vi "Test D Datagrid.vi"() -> ()   [LabVIEW 2020]
uses:
  U32 D Element/U32 D Element.lvclass
  C:/dev/D Datagrid/DatagridElement/DatagridElement.lvclass
  Float D Element/Float D Element.lvclass
  Bool D Element/Bool D Element.lvclass
  U32 D Element/Display mode.ctl
  Double D Element/Double D Element.lvclass
  C:/dev/D Datagrid/Floating point base/Floating point base.lvclass
  D_Datagrid.lvclass
  U32 D Element/U32 D Element.lvclass/U32 D Element.ctl
  Floating point base/Floating point base.lvclass/Floating point base.ctl
  D_Datagrid.lvclass/D_Datagrid.ctl
  Floating point base/Write Format string.vi
  U32 D Element/Write Display mode.vi
  Read Auto update indicator.vi
  Redraw full indicator.vi
panel:
  in  "Table Control":string[][](table)
  # "#TODO:\n\n-Make sure all keybinds work correctly (tabs?)"
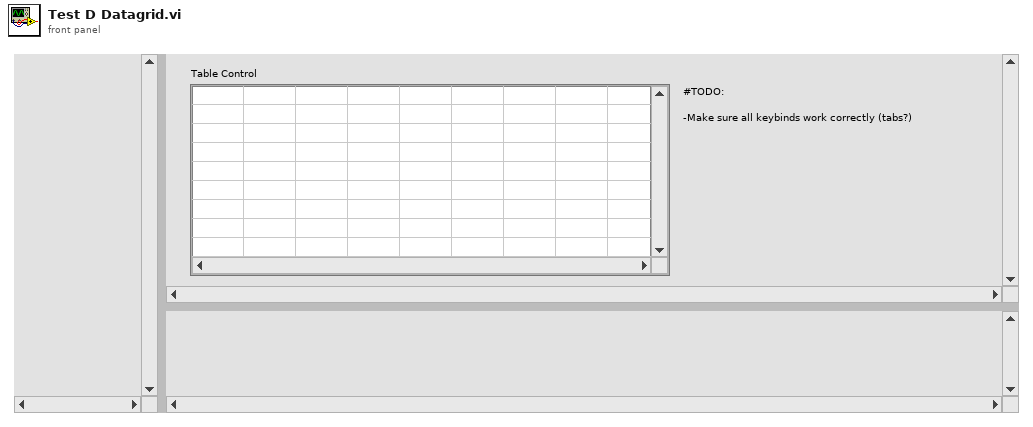
[diagram p1: front panel]
types:
  T1 = typedef "D Datagrid Library.lvlib/U32 D Element.lvclass/Display mode.ctl" = enum16{"Standard", "Hex"}
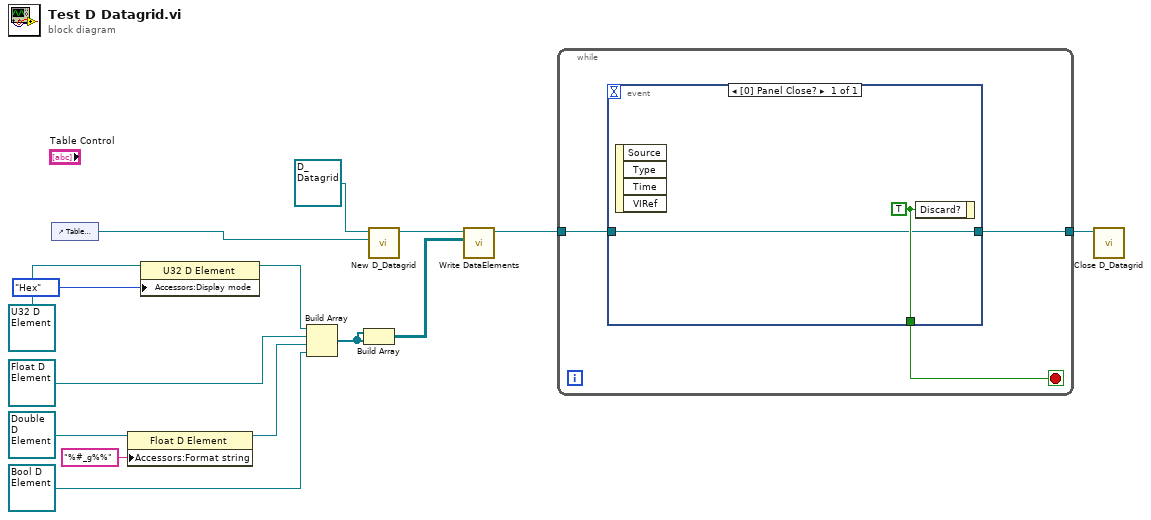
[diagram p0: block diagram]
diagram:
  n1 = control-ref of="Table Control"() -> (w15:refnum<vi>)
  n2 = property class="Float D Element"(reference=refnum<class "Double D Element.lvclass"> refnum ("D Datagrid Library.lvlib:Float D Element"), "Accessors:Format string"="%#_g%%" ("Format string")) -> (reference out=w3:refnum<class "Double D Element.lvclass">)  [unwired: 1 in, 1 out]
  n3 = property class="U32 D Element"(reference=refnum<class "U32 D Element.lvclass"> refnum ("U32 D Element.lvclass"), "Accessors:Display mode"=Display_mode."Hex" ("Display mode")) -> (reference out=w6:refnum<class "U32 D Element.lvclass">)  [unwired: 1 in, 1 out]
  n4 = Build Array(w6, refnum<class "Float D Element.lvclass"> refnum ("Float D Element.lvclass"), w3, refnum<class "Bool D Element.lvclass"> refnum ("Bool D Element.lvclass")) -> (w13:refnum<class "DatagridElement.lvclass">[])
  n5 = Build Array(w13, w13) -> (w12:refnum<class "DatagridElement.lvclass">[][])
  n6 = call-dynamic "New D_Datagrid.vi"("Indicator reference"=w15, "D_Datagrid in"=refnum<class "D_Datagrid.lvclass"> refnum) -> ("D_Datagrid out"=w11:refnum<class "D_Datagrid.lvclass">)  [unwired: 6 in, 3 out]
  n7 = call "Write DataElements.vi"("Data elements"=w12, "D_Datagrid in"=w11) -> ("D_Datagrid out"=w10:refnum<class "D_Datagrid.lvclass">)  [unwired: 8 in, 1 out]
  n8 = while {
    tunnel: [w17] -> w14
    tunnel: w10 -> [w16]
    stop <- w18 stop-if-true
    n9 = event shown="[0] Panel Close?" {
      selector: _ -> [_]
      dyn-events: _ -> [_]
      timeout: _ -> [_]
      tunnel: [w20] -> w18
      tunnel: [w19] -> w17
      tunnel: w16 -> [w19]
      event Panel Close? {
        w20 = TRUE ("Discard?")
        n10 = event-data() -> ()  [unwired: 1 in, 4 out]
        n11 = event-data("Discard?"=w20) -> ()  [unwired: 1 in, 1 out]
      }
    }
  }
  n12 = call "Close D_Datagrid.vi"("D_Datagrid in"=w14) -> ()  [unwired: 10 in, 1 out]
